vi "Stop Core.vi"(10 "final error code":i32, 11 "Manual UI in":refnum<class "Manual UI.lvclass">) -> (3 "Manual UI out":refnum<class "Manual UI.lvclass">)   [LabVIEW 2019, in "Manual UI.lvlib" / "Manual UI.lvclass"]
doc: "Call <b>Shutdown</b> then parent class stop core."
uses:
  Project/Manual UI.lvclass
  builds/Base Software/Panels/Prime Panel.lvlibp/Project/Prime Panel.lvclass
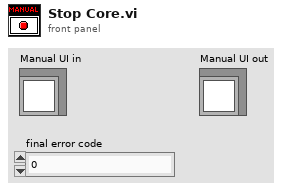
[diagram p1: front panel]
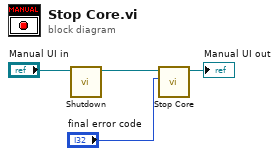
[diagram p0: block diagram]
diagram:
  n1 = call "Shutdown.vi"("Manual UI in"="Manual UI in") -> ("Manual UI out"=w1:refnum<class "Manual UI.lvclass">)  [unwired: 9 in, 1 out]
  n2 = call-parent "Stop Core.vi"("final error code"="final error code", "Monitored Actor in"=w1) -> ("Monitored Actor out"=→"Manual UI out":refnum<class "Manual UI.lvclass">)  [unwired: 9 in]
